vi "Fetch Multi Eval Meas EVM vs ChipTrace Results.vi"(7 "Result Type (Current)":i32(ring) items=["Current"=0, "Average"=1, "Maximum"=4], 8 "error in (no error)":errorcluster, 9 "Instance (1)":i32=1, 11 "VISA resource name":refnum<visa-resource-name>) -> (0 "error out":errorcluster, 1 "Reliability":i32, 2 "Results":dbl[](array[numeric]) format="%^.3e", 3 "VISA resource name out":refnum<visa-resource-name>)   [LabVIEW 2015, in "Rohde&Schwarz CMP LR WPAN Measurement.lvlib"]
doc: "Returns the offset EVM vs chip traces. One value per two chips within the PSDU is returned.\n\nAttribute:\n-\n\nRemote-control commands:\nFETCh:WPAN:MEAS<i>:MEValuation:TRACe:EVMChip[:OFFSet]:CURRent?\nFETCh:WPAN:MEAS<i>:MEValuation:TRACe:EVMChip[:OFFSet]:AVERage?\nFETCh:WPAN:MEAS<i>:MEValuation:TRACe:EVMChip[:OFFSet]:MAXimum?"
uses:
  <instrlib>/Rohde&Schwarz CMP LR WPAN Measurement/Rohde&Schwarz CMP LR WPAN Measurement.lvlib
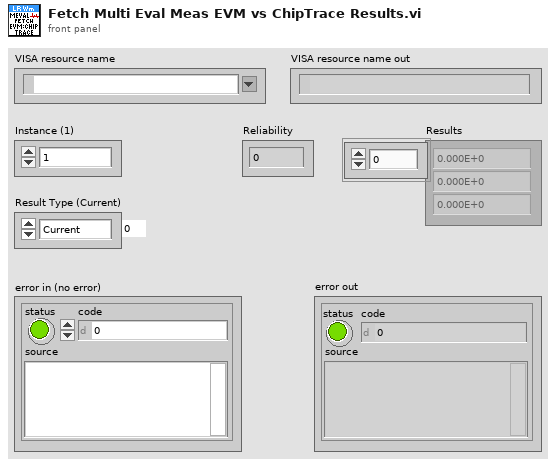
[diagram p1: front panel]
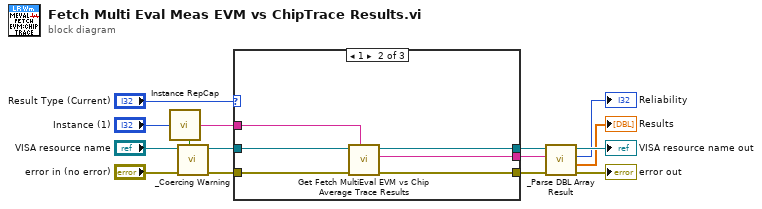
[diagram p0: block diagram]
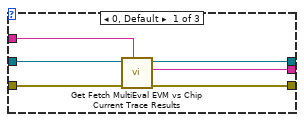
[diagram p2: hidden frame]
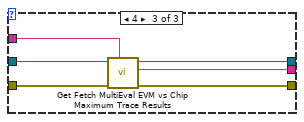
[diagram p3: hidden frame]
diagram:
  n1 = call <instrlib>:"Instance RepCap.vi"("Instance In"="Instance (1)") -> ("In Range?"=w14:bool, "RepCap Identifier Out"=w15:string)  [unwired: 1 in]
  n2 = call <instrlib>:"_Coercing Warning.vi"("In Range?"=w14, "error in (no error)"="error in (no error)", "VISA resource name"="VISA resource name") -> ("error out"=w11:errorcluster, "VISA resource name out"=w10:refnum<visa-resource-name>)  [unwired: 7 in]
  n3 = case shown="1" "Result Type (Current)" {
    tunnel: w15 -> [w21 w27 w33]
    tunnel: w10 -> [w20 w25 w31]
    tunnel: w11 -> [w19 w26 w32]
    tunnel: [w16 w22 w28] -> w5
    tunnel: [w18 w24 w30] -> w4
    tunnel: [w17 w23 w29] -> w3
    frame 0, Default {
      n4 = call "Get Fetch MultiEval EVM vs Chip Current Trace Results"("Repeated Capabilities"=w21, "error in (no error)"=w19, "instrument handle"=w20) -> ("error out"=w18:errorcluster, "Fetch MultiEval EVM vs Chip Current Trace Results"=w17:string, "instrument handle out"=w16:refnum<visa-resource-name>)  [unwired: 6 in]
    }
    frame 1 {
      n5 = call "Get Fetch MultiEval EVM vs Chip Average Trace Results"("Repeated Capabilities"=w27, "error in (no error)"=w26, "instrument handle"=w25) -> ("error out"=w24:errorcluster, "Fetch MultiEval EVM vs Chip Average Trace Results"=w23:string, "instrument handle out"=w22:refnum<visa-resource-name>)  [unwired: 6 in]
    }
    frame 4 {
      n6 = call "Get Fetch MultiEval EVM vs Chip Maximum Trace Results"("Repeated Capabilities"=w33, "error in (no error)"=w32, "instrument handle"=w31) -> ("error out"=w30:errorcluster, "Fetch MultiEval EVM vs Chip Maximum Trace Results"=w29:string, "instrument handle out"=w28:refnum<visa-resource-name>)  [unwired: 6 in]
    }
  }
  n7 = call <instrlib>:"_Parse DBL Array Result.vi"("error in (no error)"=w4, "Input String"=w3, "VISA resource name"=w5) -> ("error out"=→"error out":errorcluster, "Results"=→"Results":dbl[], "Reliability"=→"Reliability":i32, "VISA resource name out"=→"VISA resource name out":refnum<visa-resource-name>)  [unwired: 5 in]
